vi "Time_passed.vi"(8 "Global Start Time":i64, 11 "State in":T1) -> (2 "Time passed":bool, 4 "x-y":i64)   [LabVIEW 2016]
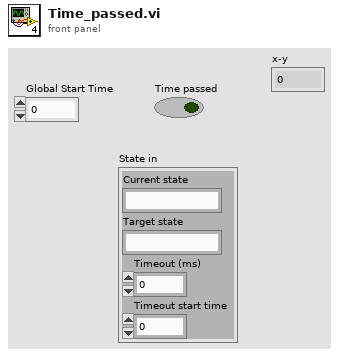
[diagram p1: front panel]
types:
  T1 = cluster{"Current state":string, "Target state":string, "Timeout (ms)":dbl, "Timeout start time":i64}
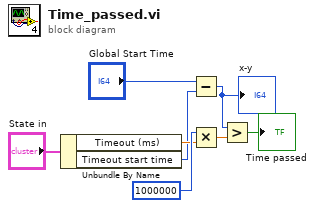
[diagram p0: block diagram]
diagram:
  n1 = Unbundle By Name("State in") -> ("Timeout (ms)"=w4:dbl, "Timeout start time"=w3:i64)
  n2 = Subtract(x="Global Start Time", y=w3) -> (x-y=w1:i64)
  "x-y" <- w1
  n3 = Multiply(x=i64 1000000 ("y"), y=w4) -> (x*y=w7:dbl)
  n4 = Greater?(x=w1, y=w7) -> (0:→"Time passed":bool)
